vi "Launch UI Thread.vi"(6 "SubPanel?(False)":bool, 7 "VI Extern Value":cluster{"Value":variant, "Key":string}[](array[cluster]), 8 "error in (no error)":errorcluster, 9 "Open?(True)":bool=TRUE, 10 "vi path":path, 11 "This VI":refnum<vi>) -> (0 "error out":errorcluster, 3 "VI Running Refnum":refnum<vi>)   [LabVIEW 2015]
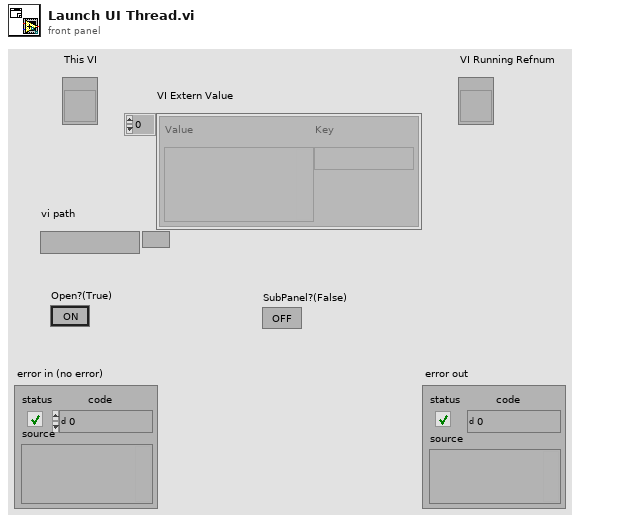
[diagram p1: front panel]
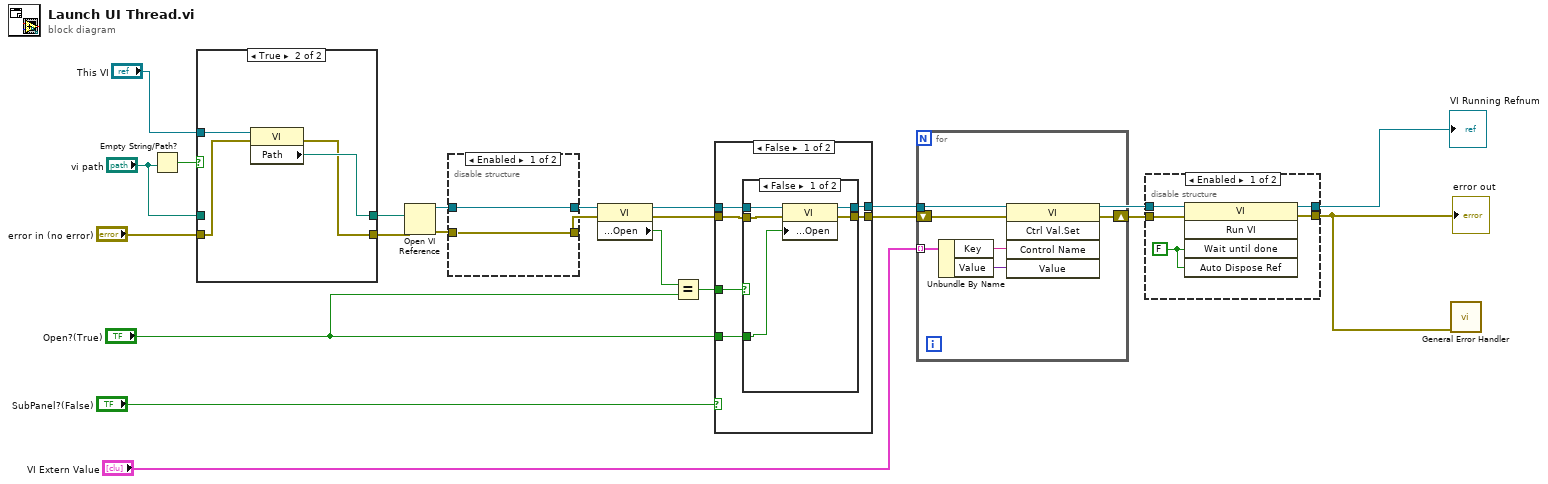
[diagram p0: block diagram]
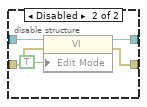
[diagram p3: hidden frame]
diagram:
  n1 = Empty String/Path?(string/path="vi path") -> (empty?=w20:bool)
  n2 = case shown="True" w20 {
    tunnel: "This VI" -> [_ w28]
    tunnel: "error in (no error)" -> [w23 w27]
    tunnel: [w24 w26] -> w16
    tunnel: "vi path" -> [w24 _]
    tunnel: [w23 w25] -> w15
    frame False {
    }
    frame True {
      n3 = property class="VI"(reference=w28, error in=w27) -> (error out=w25:errorcluster, "Path"=w26:path)  [unwired: 1 out]
    }
  }
  n4 = Open VI Reference(vi path=w16, error in (no error)=w15) -> (vi reference=w4:refnum<vi>, error out=w3:errorcluster)  [unwired: 4 in]
  n5 = disable-structure shown="Enabled" {
    disable-tunnel: w4 -> [w30 w35]
    disable-tunnel: w3 -> [w29 w34]
    disable-tunnel: [w30 w33] -> w2
    disable-tunnel: [w29 w32] -> w1
    frame Enabled {
    }
    frame Disabled {
      n6 = property class="VI"(reference=w35, error in=w34, "Edit Mode"=TRUE ("Edit Mode On Open")) -> (reference out=w33:refnum<vi>, error out=w32:errorcluster)
    }
  }
  n7 = property class="VI"(reference=w2, error in=w1) -> (reference out=w22:refnum<vi>, error out=w21:errorcluster, "Front Panel.Open"=w14:bool)
  n8 = Equal?(x=w14, y="Open?(True)") -> (x = y?=w13:bool)
  n9 = case shown="False" "SubPanel?(False)" {
    tunnel: w22 -> [w41 w50]
    tunnel: w21 -> [w40 w49]
    tunnel: w13 -> [w39 _]
    tunnel: "Open?(True)" -> [w38 _]
    tunnel: [w37 w49] -> w9
    tunnel: [w36 w50] -> w7
    frame False {
      n10 = case shown="False" w39 {
        tunnel: w41 -> [w45 w48]
        tunnel: [w46 w48] -> w36
        tunnel: w40 -> [w44 w47]
        tunnel: [w43 w47] -> w37
        tunnel: w38 -> [w42 _]
        frame False {
          n11 = property class="VI"(reference=w45, error in=w44, "Front Panel.Open"=w42) -> (reference out=w46:refnum<vi>, error out=w43:errorcluster)
        }
        frame True {
        }
      }
    }
    frame True {
    }
  }
  n12 = for {
    tunnel: w7 -> [w56]
    tunnel: "VI Extern Value" -> [w54] mode=indexing
    shift-right: [w51] -> w6
    shift-left: w9 -> [w55]
    n13 = Unbundle By Name(w54) -> ("Key"=w53:string, "Value"=w52:variant)
    n14 = invoke class="VI" method="Ctrl Val.Set"(reference=w56, error in=w55, "Control Name"=w53, "Value"=w52) -> (error out=w51:errorcluster)  [unwired: 1 in, 4 out]
  }
  n15 = disable-structure shown="Enabled" {
    disable-tunnel: [w60 w63] -> w11
    disable-tunnel: [w59 w62] -> w10
    disable-tunnel: w7 -> [w58 w63]
    disable-tunnel: w6 -> [w57 w62]
    frame Enabled {
      w61 = FALSE
      n16 = invoke class="VI" method="Run VI"(reference=w58, error in=w57, "Wait until done"=w61, "Auto Dispose Ref"=w61) -> (reference out=w60:refnum<vi>, error out=w59:errorcluster)  [unwired: 1 in, 3 out]
    }
    frame Disabled {
    }
  }
  "error out" <- w10
  "VI Running Refnum" <- w11
  n17 = call <vilib>:"General Error Handler.vi"("error in (no error)"=w10) -> ()  [unwired: 10 in, 5 out]
